vi "Viterbi.vi"(7 "Кадр с мягкими\nзначениями":dbl[](array[numeric])) -> (8 "Декодированный поток битов":bool[](array[boolean]))   [LabVIEW 2017]
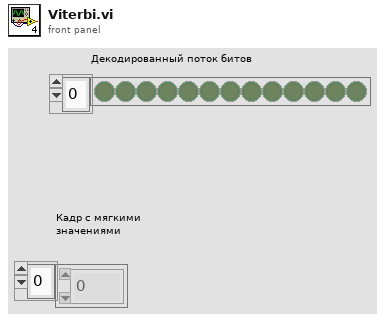
[diagram p1: front panel]
types:
  T1 = cluster{"Пр сост0":i32, "Ном зн\nреб0":i32, "Пр сост1":i32, "Ном зн\nреб1":i32, "Бит":bool}[]
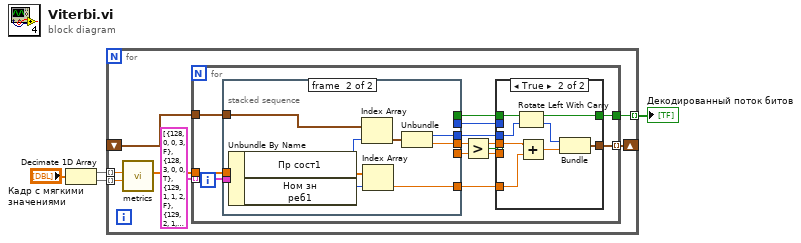
[diagram p0: block diagram]
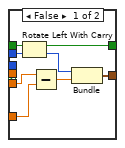
[diagram p2: hidden frame]
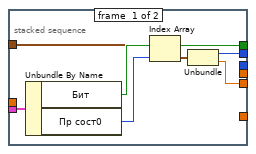
[diagram p3: hidden frame]
diagram:
  n1 = Decimate 1D Array("Кадр с мягкими\nзначениями") -> (w2:dbl[], w1:dbl[])
  n2 = for {
    tunnel: w2 -> [w10] mode=indexing
    tunnel: w1 -> [w9] mode=indexing
    tunnel: [w6] -> w3 mode=indexing
    shift-right: [w7] -> _
    shift-left: _ -> [w5]
    n3 = call "metrics.vi"("Бит неч"=w9, "Бит чет"=w10) -> ("Возможные\nметрики ребер"=w11:dbl[])  [unwired: 9 in]
    n4 = for {
      tunnel: T1 [{"Пр сост0"=128, "Ном зн\nреб0"=0, "Пр сост1"=0, "Ном зн\nреб1"=3, "Бит"=FALSE}, {"Пр сост0"=128, "Ном зн\nреб0"=3, "Пр сост1"=0, "Ном зн\nреб1"=0, "Бит"=TRUE}, {"Пр сост0"=129, "Ном зн\nреб0"=1, "Пр сост1"=1, "Ном зн\nреб1"=2, "Бит"=FALSE}, {"Пр сост0"=129, "Ном зн\nреб0"=2, "Пр сост1"=1, "Ном зн\nреб1"=1, "Бит"=TRUE}, {"Пр сост0"=130, "Ном зн\nреб0"=3, "Пр сост1"=2, "Ном зн\nреб1"=0, "Бит"=FALSE}, {"Пр сост0"=130, "Ном зн\nреб0"=0, "Пр сост1"=2, "Ном зн\nреб1"=3, "Бит"=TRUE}, {"Пр сост0"=131, "Ном зн\nреб0"=2, "Пр сост1"=3, "Ном зн\nреб1"=1, "Бит"=FALSE}, {"Пр сост0"=131, "Ном зн\nреб0"=1, "Пр сост1"=3, "Ном зн\nреб1"=2, "Бит"=TRUE}, {"Пр сост0"=132, "Ном зн\nреб0"=3, "Пр сост1"=4, "Ном зн\nреб1"=0, "Бит"=FALSE}, {"Пр сост0"=132, "Ном зн\nреб0"=0, "Пр сост1"=4, "Ном зн\nреб1"=3, "Бит"=TRUE}, {"Пр сост0"=133, "Ном зн\nреб0"=2, "Пр сост1"=5, "Ном зн\nреб1"=1, "Бит"=FALSE}, {"Пр сост0"=133, "Ном зн\nреб0"=1, "Пр сост1"=5, "Ном зн\nреб1"=2, "Бит"=TRUE}, {"Пр сост0"=134, "Ном зн\nреб0"=0, "Пр сост1"=6, "Ном зн\nреб1"=3, "Бит"=FALSE}, {"Пр сост0"=134, "Ном зн\nреб0"=3, "Пр сост1"=6, "Ном зн\nреб1"=0, "Бит"=TRUE}, {"Пр сост0"=135, "Ном зн\nреб0"=1, "Пр сост1"=7, "Ном зн\nреб1"=2, "Бит"=FALSE}, {"Пр сост0"=135, "Ном зн\nреб0"=2, "Пр сост1"=7, "Ном зн\nреб1"=1, "Бит"=TRUE}, {"Пр сост0"=136, "Ном зн\nреб0"=2, "Пр сост1"=8, "Ном зн\nреб1"=1, "Бит"=FALSE}, {"Пр сост0"=136, "Ном зн\nреб0"=1, "Пр сост1"=8, "Ном зн\nреб1"=2, "Бит"=TRUE}, {"Пр сост0"=137, "Ном зн\nреб0"=3, "Пр сост1"=9, "Ном зн\nреб1"=0, "Бит"=FALSE}, {"Пр сост0"=137, "Ном зн\nреб0"=0, "Пр сост1"=9, "Ном зн\nреб1"=3, "Бит"=TRUE}, {"Пр сост0"=138, "Ном зн\nреб0"=1, "Пр сост1"=10, "Ном зн\nреб1"=2, "Бит"=FALSE}, {"Пр сост0"=138, "Ном зн\nреб0"=2, "Пр сост1"=10, "Ном зн\nреб1"=1, "Бит"=TRUE}, {"Пр сост0"=139, "Ном зн\nреб0"=0, "Пр сост1"=11, "Ном зн\nреб1"=3, "Бит"=FALSE}, {"Пр сост0"=139, "Ном зн\nреб0"=3, "Пр сост1"=11, "Ном зн\nреб1"=0, "Бит"=TRUE}, {"Пр сост0"=140, "Ном зн\nреб0"=1, "Пр сост1"=12, "Ном зн\nреб1"=2, "Бит"=FALSE}, {"Пр сост0"=140, "Ном зн\nреб0"=2, "Пр сост1"=12, "Ном зн\nреб1"=1, "Бит"=TRUE}, {"Пр сост0"=141, "Ном зн\nреб0"=0, "Пр сост1"=13, "Ном зн\nреб1"=3, "Бит"=FALSE}, {"Пр сост0"=141, "Ном зн\nреб0"=3, "Пр сост1"=13, "Ном зн\nреб1"=0, "Бит"=TRUE}, {"Пр сост0"=142, "Ном зн\nреб0"=2, "Пр сост1"=14, "Ном зн\nреб1"=1, "Бит"=FALSE}, {"Пр сост0"=142, "Ном зн\nреб0"=1, "Пр сост1"=14, "Ном зн\nреб1"=2, "Бит"=TRUE}, {"Пр сост0"=143, "Ном зн\nреб0"=3, "Пр сост1"=15, "Ном зн\nреб1"=0, "Бит"=FALSE}, {"Пр сост0"=143, "Ном зн\nреб0"=0, "Пр сост1"=15, "Ном зн\nреб1"=3, "Бит"=TRUE}, {"Пр сост0"=144, "Ном зн\nреб0"=1, "Пр сост1"=16, "Ном зн\nреб1"=2, "Бит"=FALSE}, {"Пр сост0"=144, "Ном зн\nреб0"=2, "Пр сост1"=16, "Ном зн\nреб1"=1, "Бит"=TRUE}, {"Пр сост0"=145, "Ном зн\nреб0"=0, "Пр сост1"=17, "Ном зн\nреб1"=3, "Бит"=FALSE}, {"Пр сост0"=145, "Ном зн\nреб0"=3, "Пр сост1"=17, "Ном зн\nреб1"=0, "Бит"=TRUE}, {"Пр сост0"=146, "Ном зн\nреб0"=2, "Пр сост1"=18, "Ном зн\nреб1"=1, "Бит"=FALSE}, {"Пр сост0"=146, "Ном зн\nреб0"=1, "Пр сост1"=18, "Ном зн\nреб1"=2, "Бит"=TRUE}, {"Пр сост0"=147, "Ном зн\nреб0"=3, "Пр сост1"=19, "Ном зн\nреб1"=0, "Бит"=FALSE}, {"Пр сост0"=147, "Ном зн\nреб0"=0, "Пр сост1"=19, "Ном зн\nреб1"=3, "Бит"=TRUE}, {"Пр сост0"=148, "Ном зн\nреб0"=2, "Пр сост1"=20, "Ном зн\nреб1"=1, "Бит"=FALSE}, {"Пр сост0"=148, "Ном зн\nреб0"=1, "Пр сост1"=20, "Ном зн\nреб1"=2, "Бит"=TRUE}, {"Пр сост0"=149, "Ном зн\nреб0"=3, "Пр сост1"=21, "Ном зн\nреб1"=0, "Бит"=FALSE}, {"Пр сост0"=149, "Ном зн\nреб0"=0, "Пр сост1"=21, "Ном зн\nреб1"=3, "Бит"=TRUE}, {"Пр сост0"=150, "Ном зн\nреб0"=1, "Пр сост1"=22, "Ном зн\nреб1"=2, "Бит"=FALSE}, {"Пр сост0"=150, "Ном зн\nреб0"=2, "Пр сост1"=22, "Ном зн\nреб1"=1, "Бит"=TRUE}, {"Пр сост0"=151, "Ном зн\nреб0"=0, "Пр сост1"=23, "Ном зн\nреб1"=3, "Бит"=FALSE}, {"Пр сост0"=151, "Ном зн\nреб0"=3, "Пр сост1"=23, "Ном зн\nреб1"=0, "Бит"=TRUE}, {"Пр сост0"=152, "Ном зн\nреб0"=3, "Пр сост1"=24, "Ном зн\nреб1"=0, "Бит"=FALSE}, {"Пр сост0"=152, "Ном зн\nреб0"=0, "Пр сост1"=24, "Ном зн\nреб1"=3, "Бит"=TRUE}, {"Пр сост0"=153, "Ном зн\nреб0"=2, "Пр сост1"=25, "Ном зн\nреб1"=1, "Бит"=FALSE}, {"Пр сост0"=153, "Ном зн\nреб0"=1, "Пр сост1"=25, "Ном зн\nреб1"=2, "Бит"=TRUE}, {"Пр сост0"=154, "Ном зн\nреб0"=0, "Пр сост1"=26, "Ном зн\nреб1"=3, "Бит"=FALSE}, {"Пр сост0"=154, "Ном зн\nреб0"=3, "Пр сост1"=26, "Ном зн\nреб1"=0, "Бит"=TRUE}, {"Пр сост0"=155, "Ном зн\nреб0"=1, "Пр сост1"=27, "Ном зн\nреб1"=2, "Бит"=FALSE}, {"Пр сост0"=155, "Ном зн\nреб0"=2, "Пр сост1"=27, "Ном зн\nреб1"=1, "Бит"=TRUE}, {"Пр сост0"=156, "Ном зн\nреб0"=0, "Пр сост1"=28, "Ном зн\nреб1"=3, "Бит"=FALSE}, {"Пр сост0"=156, "Ном зн\nреб0"=3, "Пр сост1"=28, "Ном зн\nреб1"=0, "Бит"=TRUE}, {"Пр сост0"=157, "Ном зн\nреб0"=1, "Пр сост1"=29, "Ном зн\nреб1"=2, "Бит"=FALSE}, {"Пр сост0"=157, "Ном зн\nреб0"=2, "Пр сост1"=29, "Ном зн\nреб1"=1, "Бит"=TRUE}, {"Пр сост0"=158, "Ном зн\nреб0"=3, "Пр сост1"=30, "Ном зн\nреб1"=0, "Бит"=FALSE}, {"Пр сост0"=158, "Ном зн\nреб0"=0, "Пр сост1"=30, "Ном зн\nреб1"=3, "Бит"=TRUE}, {"Пр сост0"=159, "Ном зн\nреб0"=2, "Пр сост1"=31, "Ном зн\nреб1"=1, "Бит"=FALSE}, {"Пр сост0"=159, "Ном зн\nреб0"=1, "Пр сост1"=31, "Ном зн\nреб1"=2, "Бит"=TRUE}, {"Пр сост0"=160, "Ном зн\nреб0"=0, "Пр сост1"=32, "Ном зн\nреб1"=3, "Бит"=FALSE}, {"Пр сост0"=160, "Ном зн\nреб0"=3, "Пр сост1"=32, "Ном зн\nреб1"=0, "Бит"=TRUE}, {"Пр сост0"=161, "Ном зн\nреб0"=1, "Пр сост1"=33, "Ном зн\nреб1"=2, "Бит"=FALSE}, {"Пр сост0"=161, "Ном зн\nреб0"=2, "Пр сост1"=33, "Ном зн\nреб1"=1, "Бит"=TRUE}, {"Пр сост0"=162, "Ном зн\nреб0"=3, "Пр сост1"=34, "Ном зн\nреб1"=0, "Бит"=FALSE}, {"Пр сост0"=162, "Ном зн\nреб0"=0, "Пр сост1"=34, "Ном зн\nреб1"=3, "Бит"=TRUE}, {"Пр сост0"=163, "Ном зн\nреб0"=2, "Пр сост1"=35, "Ном зн\nреб1"=1, "Бит"=FALSE}, {"Пр сост0"=163, "Ном зн\nреб0"=1, "Пр сост1"=35, "Ном зн\nреб1"=2, "Бит"=TRUE}, {"Пр сост0"=164, "Ном зн\nреб0"=3, "Пр сост1"=36, "Ном зн\nреб1"=0, "Бит"=FALSE}, {"Пр сост0"=164, "Ном зн\nреб0"=0, "Пр сост1"=36, "Ном зн\nреб1"=3, "Бит"=TRUE}, {"Пр сост0"=165, "Ном зн\nреб0"=2, "Пр сост1"=37, "Ном зн\nреб1"=1, "Бит"=FALSE}, {"Пр сост0"=165, "Ном зн\nреб0"=1, "Пр сост1"=37, "Ном зн\nреб1"=2, "Бит"=TRUE}, {"Пр сост0"=166, "Ном зн\nреб0"=0, "Пр сост1"=38, "Ном зн\nреб1"=3, "Бит"=FALSE}, {"Пр сост0"=166, "Ном зн\nреб0"=3, "Пр сост1"=38, "Ном зн\nреб1"=0, "Бит"=TRUE}, {"Пр сост0"=167, "Ном зн\nреб0"=1, "Пр сост1"=39, "Ном зн\nреб1"=2, "Бит"=FALSE}, {"Пр сост0"=167, "Ном зн\nреб0"=2, "Пр сост1"=39, "Ном зн\nреб1"=1, "Бит"=TRUE}, {"Пр сост0"=168, "Ном зн\nреб0"=2, "Пр сост1"=40, "Ном зн\nреб1"=1, "Бит"=FALSE}, {"Пр сост0"=168, "Ном зн\nреб0"=1, "Пр сост1"=40, "Ном зн\nреб1"=2, "Бит"=TRUE}, {"Пр сост0"=169, "Ном зн\nреб0"=3, "Пр сост1"=41, "Ном зн\nреб1"=0, "Бит"=FALSE}, {"Пр сост0"=169, "Ном зн\nреб0"=0, "Пр сост1"=41, "Ном зн\nреб1"=3, "Бит"=TRUE}, {"Пр сост0"=170, "Ном зн\nреб0"=1, "Пр сост1"=42, "Ном зн\nреб1"=2, "Бит"=FALSE}, {"Пр сост0"=170, "Ном зн\nреб0"=2, "Пр сост1"=42, "Ном зн\nреб1"=1, "Бит"=TRUE}, {"Пр сост0"=171, "Ном зн\nреб0"=0, "Пр сост1"=43, "Ном зн\nреб1"=3, "Бит"=FALSE}, {"Пр сост0"=171, "Ном зн\nреб0"=3, "Пр сост1"=43, "Ном зн\nреб1"=0, "Бит"=TRUE}, {"Пр сост0"=172, "Ном зн\nреб0"=1, "Пр сост1"=44, "Ном зн\nреб1"=2, "Бит"=FALSE}, {"Пр сост0"=172, "Ном зн\nреб0"=2, "Пр сост1"=44, "Ном зн\nреб1"=1, "Бит"=TRUE}, {"Пр сост0"=173, "Ном зн\nреб0"=0, "Пр сост1"=45, "Ном зн\nреб1"=3, "Бит"=FALSE}, {"Пр сост0"=173, "Ном зн\nреб0"=3, "Пр сост1"=45, "Ном зн\nреб1"=0, "Бит"=TRUE}, {"Пр сост0"=174, "Ном зн\nреб0"=2, "Пр сост1"=46, "Ном зн\nреб1"=1, "Бит"=FALSE}, {"Пр сост0"=174, "Ном зн\nреб0"=1, "Пр сост1"=46, "Ном зн\nреб1"=2, "Бит"=TRUE}, {"Пр сост0"=175, "Ном зн\nреб0"=3, "Пр сост1"=47, "Ном зн\nреб1"=0, "Бит"=FALSE}, {"Пр сост0"=175, "Ном зн\nреб0"=0, "Пр сост1"=47, "Ном зн\nреб1"=3, "Бит"=TRUE}, {"Пр сост0"=176, "Ном зн\nреб0"=1, "Пр сост1"=48, "Ном зн\nреб1"=2, "Бит"=FALSE}, {"Пр сост0"=176, "Ном зн\nреб0"=2, "Пр сост1"=48, "Ном зн\nреб1"=1, "Бит"=TRUE}, {"Пр сост0"=177, "Ном зн\nреб0"=0, "Пр сост1"=49, "Ном зн\nреб1"=3, "Бит"=FALSE}, {"Пр сост0"=177, "Ном зн\nреб0"=3, "Пр сост1"=49, "Ном зн\nреб1"=0, "Бит"=TRUE}, {"Пр сост0"=178, "Ном зн\nреб0"=2, "Пр сост1"=50, "Ном зн\nреб1"=1, "Бит"=FALSE}, {"Пр сост0"=178, "Ном зн\nреб0"=1, "Пр сост1"=50, "Ном зн\nреб1"=2, "Бит"=TRUE}, {"Пр сост0"=179, "Ном зн\nреб0"=3, "Пр сост1"=51, "Ном зн\nреб1"=0, "Бит"=FALSE}, {"Пр сост0"=179, "Ном зн\nреб0"=0, "Пр сост1"=51, "Ном зн\nреб1"=3, "Бит"=TRUE}, {"Пр сост0"=180, "Ном зн\nреб0"=2, "Пр сост1"=52, "Ном зн\nреб1"=1, "Бит"=FALSE}, {"Пр сост0"=180, "Ном зн\nреб0"=1, "Пр сост1"=52, "Ном зн\nреб1"=2, "Бит"=TRUE}, {"Пр сост0"=181, "Ном зн\nреб0"=3, "Пр сост1"=53, "Ном зн\nреб1"=0, "Бит"=FALSE}, {"Пр сост0"=181, "Ном зн\nреб0"=0, "Пр сост1"=53, "Ном зн\nреб1"=3, "Бит"=TRUE}, {"Пр сост0"=182, "Ном зн\nреб0"=1, "Пр сост1"=54, "Ном зн\nреб1"=2, "Бит"=FALSE}, {"Пр сост0"=182, "Ном зн\nреб0"=2, "Пр сост1"=54, "Ном зн\nреб1"=1, "Бит"=TRUE}, {"Пр сост0"=183, "Ном зн\nреб0"=0, "Пр сост1"=55, "Ном зн\nреб1"=3, "Бит"=FALSE}, {"Пр сост0"=183, "Ном зн\nреб0"=3, "Пр сост1"=55, "Ном зн\nреб1"=0, "Бит"=TRUE}, {"Пр сост0"=184, "Ном зн\nреб0"=3, "Пр сост1"=56, "Ном зн\nреб1"=0, "Бит"=FALSE}, {"Пр сост0"=184, "Ном зн\nреб0"=0, "Пр сост1"=56, "Ном зн\nреб1"=3, "Бит"=TRUE}, {"Пр сост0"=185, "Ном зн\nреб0"=2, "Пр сост1"=57, "Ном зн\nреб1"=1, "Бит"=FALSE}, {"Пр сост0"=185, "Ном зн\nреб0"=1, "Пр сост1"=57, "Ном зн\nреб1"=2, "Бит"=TRUE}, {"Пр сост0"=186, "Ном зн\nреб0"=0, "Пр сост1"=58, "Ном зн\nреб1"=3, "Бит"=FALSE}, {"Пр сост0"=186, "Ном зн\nреб0"=3, "Пр сост1"=58, "Ном зн\nреб1"=0, "Бит"=TRUE}, {"Пр сост0"=187, "Ном зн\nреб0"=1, "Пр сост1"=59, "Ном зн\nреб1"=2, "Бит"=FALSE}, {"Пр сост0"=187, "Ном зн\nреб0"=2, "Пр сост1"=59, "Ном зн\nреб1"=1, "Бит"=TRUE}, {"Пр сост0"=188, "Ном зн\nреб0"=0, "Пр сост1"=60, "Ном зн\nреб1"=3, "Бит"=FALSE}, {"Пр сост0"=188, "Ном зн\nреб0"=3, "Пр сост1"=60, "Ном зн\nреб1"=0, "Бит"=TRUE}, {"Пр сост0"=189, "Ном зн\nреб0"=1, "Пр сост1"=61, "Ном зн\nреб1"=2, "Бит"=FALSE}, {"Пр сост0"=189, "Ном зн\nреб0"=2, "Пр сост1"=61, "Ном зн\nреб1"=1, "Бит"=TRUE}, {"Пр сост0"=190, "Ном зн\nреб0"=3, "Пр сост1"=62, "Ном зн\nреб1"=0, "Бит"=FALSE}, {"Пр сост0"=190, "Ном зн\nреб0"=0, "Пр сост1"=62, "Ном зн\nреб1"=3, "Бит"=TRUE}, {"Пр сост0"=191, "Ном зн\nреб0"=2, "Пр сост1"=63, "Ном зн\nреб1"=1, "Бит"=FALSE}, {"Пр сост0"=191, "Ном зн\nреб0"=1, "Пр сост1"=63, "Ном зн\nреб1"=2, "Бит"=TRUE}, {"Пр сост0"=192, "Ном зн\nреб0"=1, "Пр сост1"=64, "Ном зн\nреб1"=2, "Бит"=FALSE}, {"Пр сост0"=192, "Ном зн\nреб0"=2, "Пр сост1"=64, "Ном зн\nреб1"=1, "Бит"=TRUE}, {"Пр сост0"=193, "Ном зн\nреб0"=0, "Пр сост1"=65, "Ном зн\nреб1"=3, "Бит"=FALSE}, {"Пр сост0"=193, "Ном зн\nреб0"=3, "Пр сост1"=65, "Ном зн\nреб1"=0, "Бит"=TRUE}, {"Пр сост0"=194, "Ном зн\nреб0"=2, "Пр сост1"=66, "Ном зн\nреб1"=1, "Бит"=FALSE}, {"Пр сост0"=194, "Ном зн\nреб0"=1, "Пр сост1"=66, "Ном зн\nреб1"=2, "Бит"=TRUE}, {"Пр сост0"=195, "Ном зн\nреб0"=3, "Пр сост1"=67, "Ном зн\nреб1"=0, "Бит"=FALSE}, {"Пр сост0"=195, "Ном зн\nреб0"=0, "Пр сост1"=67, "Ном зн\nреб1"=3, "Бит"=TRUE}, {"Пр сост0"=196, "Ном зн\nреб0"=2, "Пр сост1"=68, "Ном зн\nреб1"=1, "Бит"=FALSE}, {"Пр сост0"=196, "Ном зн\nреб0"=1, "Пр сост1"=68, "Ном зн\nреб1"=2, "Бит"=TRUE}, {"Пр сост0"=197, "Ном зн\nреб0"=3, "Пр сост1"=69, "Ном зн\nреб1"=0, "Бит"=FALSE}, {"Пр сост0"=197, "Ном зн\nреб0"=0, "Пр сост1"=69, "Ном зн\nреб1"=3, "Бит"=TRUE}, {"Пр сост0"=198, "Ном зн\nреб0"=1, "Пр сост1"=70, "Ном зн\nреб1"=2, "Бит"=FALSE}, {"Пр сост0"=198, "Ном зн\nреб0"=2, "Пр сост1"=70, "Ном зн\nреб1"=1, "Бит"=TRUE}, {"Пр сост0"=199, "Ном зн\nреб0"=0, "Пр сост1"=71, "Ном зн\nреб1"=3, "Бит"=FALSE}, {"Пр сост0"=199, "Ном зн\nреб0"=3, "Пр сост1"=71, "Ном зн\nреб1"=0, "Бит"=TRUE}, {"Пр сост0"=200, "Ном зн\nреб0"=3, "Пр сост1"=72, "Ном зн\nреб1"=0, "Бит"=FALSE}, {"Пр сост0"=200, "Ном зн\nреб0"=0, "Пр сост1"=72, "Ном зн\nреб1"=3, "Бит"=TRUE}, {"Пр сост0"=201, "Ном зн\nреб0"=2, "Пр сост1"=73, "Ном зн\nреб1"=1, "Бит"=FALSE}, {"Пр сост0"=201, "Ном зн\nреб0"=1, "Пр сост1"=73, "Ном зн\nреб1"=2, "Бит"=TRUE}, {"Пр сост0"=202, "Ном зн\nреб0"=0, "Пр сост1"=74, "Ном зн\nреб1"=3, "Бит"=FALSE}, {"Пр сост0"=202, "Ном зн\nреб0"=3, "Пр сост1"=74, "Ном зн\nреб1"=0, "Бит"=TRUE}, {"Пр сост0"=203, "Ном зн\nреб0"=1, "Пр сост1"=75, "Ном зн\nреб1"=2, "Бит"=FALSE}, {"Пр сост0"=203, "Ном зн\nреб0"=2, "Пр сост1"=75, "Ном зн\nреб1"=1, "Бит"=TRUE}, {"Пр сост0"=204, "Ном зн\nреб0"=0, "Пр сост1"=76, "Ном зн\nреб1"=3, "Бит"=FALSE}, {"Пр сост0"=204, "Ном зн\nреб0"=3, "Пр сост1"=76, "Ном зн\nреб1"=0, "Бит"=TRUE}, {"Пр сост0"=205, "Ном зн\nреб0"=1, "Пр сост1"=77, "Ном зн\nреб1"=2, "Бит"=FALSE}, {"Пр сост0"=205, "Ном зн\nреб0"=2, "Пр сост1"=77, "Ном зн\nреб1"=1, "Бит"=TRUE}, {"Пр сост0"=206, "Ном зн\nреб0"=3, "Пр сост1"=78, "Ном зн\nреб1"=0, "Бит"=FALSE}, {"Пр сост0"=206, "Ном зн\nреб0"=0, "Пр сост1"=78, "Ном зн\nреб1"=3, "Бит"=TRUE}, {"Пр сост0"=207, "Ном зн\nреб0"=2, "Пр сост1"=79, "Ном зн\nреб1"=1, "Бит"=FALSE}, {"Пр сост0"=207, "Ном зн\nреб0"=1, "Пр сост1"=79, "Ном зн\nреб1"=2, "Бит"=TRUE}, {"Пр сост0"=208, "Ном зн\nреб0"=0, "Пр сост1"=80, "Ном зн\nреб1"=3, "Бит"=FALSE}, {"Пр сост0"=208, "Ном зн\nреб0"=3, "Пр сост1"=80, "Ном зн\nреб1"=0, "Бит"=TRUE}, {"Пр сост0"=209, "Ном зн\nреб0"=1, "Пр сост1"=81, "Ном зн\nреб1"=2, "Бит"=FALSE}, {"Пр сост0"=209, "Ном зн\nреб0"=2, "Пр сост1"=81, "Ном зн\nреб1"=1, "Бит"=TRUE}, {"Пр сост0"=210, "Ном зн\nреб0"=3, "Пр сост1"=82, "Ном зн\nреб1"=0, "Бит"=FALSE}, {"Пр сост0"=210, "Ном зн\nреб0"=0, "Пр сост1"=82, "Ном зн\nреб1"=3, "Бит"=TRUE}, {"Пр сост0"=211, "Ном зн\nреб0"=2, "Пр сост1"=83, "Ном зн\nреб1"=1, "Бит"=FALSE}, {"Пр сост0"=211, "Ном зн\nреб0"=1, "Пр сост1"=83, "Ном зн\nреб1"=2, "Бит"=TRUE}, {"Пр сост0"=212, "Ном зн\nреб0"=3, "Пр сост1"=84, "Ном зн\nреб1"=0, "Бит"=FALSE}, {"Пр сост0"=212, "Ном зн\nреб0"=0, "Пр сост1"=84, "Ном зн\nреб1"=3, "Бит"=TRUE}, {"Пр сост0"=213, "Ном зн\nреб0"=2, "Пр сост1"=85, "Ном зн\nреб1"=1, "Бит"=FALSE}, {"Пр сост0"=213, "Ном зн\nреб0"=1, "Пр сост1"=85, "Ном зн\nреб1"=2, "Бит"=TRUE}, {"Пр сост0"=214, "Ном зн\nреб0"=0, "Пр сост1"=86, "Ном зн\nреб1"=3, "Бит"=FALSE}, {"Пр сост0"=214, "Ном зн\nреб0"=3, "Пр сост1"=86, "Ном зн\nреб1"=0, "Бит"=TRUE}, {"Пр сост0"=215, "Ном зн\nреб0"=1, "Пр сост1"=87, "Ном зн\nреб1"=2, "Бит"=FALSE}, {"Пр сост0"=215, "Ном зн\nреб0"=2, "Пр сост1"=87, "Ном зн\nреб1"=1, "Бит"=TRUE}, {"Пр сост0"=216, "Ном зн\nреб0"=2, "Пр сост1"=88, "Ном зн\nреб1"=1, "Бит"=FALSE}, {"Пр сост0"=216, "Ном зн\nреб0"=1, "Пр сост1"=88, "Ном зн\nреб1"=2, "Бит"=TRUE}, {"Пр сост0"=217, "Ном зн\nреб0"=3, "Пр сост1"=89, "Ном зн\nреб1"=0, "Бит"=FALSE}, {"Пр сост0"=217, "Ном зн\nреб0"=0, "Пр сост1"=89, "Ном зн\nреб1"=3, "Бит"=TRUE}, {"Пр сост0"=218, "Ном зн\nреб0"=1, "Пр сост1"=90, "Ном зн\nреб1"=2, "Бит"=FALSE}, {"Пр сост0"=218, "Ном зн\nреб0"=2, "Пр сост1"=90, "Ном зн\nреб1"=1, "Бит"=TRUE}, {"Пр сост0"=219, "Ном зн\nреб0"=0, "Пр сост1"=91, "Ном зн\nреб1"=3, "Бит"=FALSE}, {"Пр сост0"=219, "Ном зн\nреб0"=3, "Пр сост1"=91, "Ном зн\nреб1"=0, "Бит"=TRUE}, {"Пр сост0"=220, "Ном зн\nреб0"=1, "Пр сост1"=92, "Ном зн\nреб1"=2, "Бит"=FALSE}, {"Пр сост0"=220, "Ном зн\nреб0"=2, "Пр сост1"=92, "Ном зн\nреб1"=1, "Бит"=TRUE}, {"Пр сост0"=221, "Ном зн\nреб0"=0, "Пр сост1"=93, "Ном зн\nреб1"=3, "Бит"=FALSE}, {"Пр сост0"=221, "Ном зн\nреб0"=3, "Пр сост1"=93, "Ном зн\nреб1"=0, "Бит"=TRUE}, {"Пр сост0"=222, "Ном зн\nреб0"=2, "Пр сост1"=94, "Ном зн\nреб1"=1, "Бит"=FALSE}, {"Пр сост0"=222, "Ном зн\nреб0"=1, "Пр сост1"=94, "Ном зн\nреб1"=2, "Бит"=TRUE}, {"Пр сост0"=223, "Ном зн\nреб0"=3, "Пр сост1"=95, "Ном зн\nреб1"=0, "Бит"=FALSE}, {"Пр сост0"=223, "Ном зн\nреб0"=0, "Пр сост1"=95, "Ном зн\nреб1"=3, "Бит"=TRUE}, {"Пр сост0"=224, "Ном зн\nреб0"=1, "Пр сост1"=96, "Ном зн\nреб1"=2, "Бит"=FALSE}, {"Пр сост0"=224, "Ном зн\nреб0"=2, "Пр сост1"=96, "Ном зн\nреб1"=1, "Бит"=TRUE}, {"Пр сост0"=225, "Ном зн\nреб0"=0, "Пр сост1"=97, "Ном зн\nреб1"=3, "Бит"=FALSE}, {"Пр сост0"=225, "Ном зн\nреб0"=3, "Пр сост1"=97, "Ном зн\nреб1"=0, "Бит"=TRUE}, {"Пр сост0"=226, "Ном зн\nреб0"=2, "Пр сост1"=98, "Ном зн\nреб1"=1, "Бит"=FALSE}, {"Пр сост0"=226, "Ном зн\nреб0"=1, "Пр сост1"=98, "Ном зн\nреб1"=2, "Бит"=TRUE}, {"Пр сост0"=227, "Ном зн\nреб0"=3, "Пр сост1"=99, "Ном зн\nреб1"=0, "Бит"=FALSE}, {"Пр сост0"=227, "Ном зн\nреб0"=0, "Пр сост1"=99, "Ном зн\nреб1"=3, "Бит"=TRUE}, {"Пр сост0"=228, "Ном зн\nреб0"=2, "Пр сост1"=100, "Ном зн\nреб1"=1, "Бит"=FALSE}, {"Пр сост0"=228, "Ном зн\nреб0"=1, "Пр сост1"=100, "Ном зн\nреб1"=2, "Бит"=TRUE}, {"Пр сост0"=229, "Ном зн\nреб0"=3, "Пр сост1"=101, "Ном зн\nреб1"=0, "Бит"=FALSE}, {"Пр сост0"=229, "Ном зн\nреб0"=0, "Пр сост1"=101, "Ном зн\nреб1"=3, "Бит"=TRUE}, {"Пр сост0"=230, "Ном зн\nреб0"=1, "Пр сост1"=102, "Ном зн\nреб1"=2, "Бит"=FALSE}, {"Пр сост0"=230, "Ном зн\nреб0"=2, "Пр сост1"=102, "Ном зн\nреб1"=1, "Бит"=TRUE}, {"Пр сост0"=231, "Ном зн\nреб0"=0, "Пр сост1"=103, "Ном зн\nреб1"=3, "Бит"=FALSE}, {"Пр сост0"=231, "Ном зн\nреб0"=3, "Пр сост1"=103, "Ном зн\nреб1"=0, "Бит"=TRUE}, {"Пр сост0"=232, "Ном зн\nреб0"=3, "Пр сост1"=104, "Ном зн\nреб1"=0, "Бит"=FALSE}, {"Пр сост0"=232, "Ном зн\nреб0"=0, "Пр сост1"=104, "Ном зн\nреб1"=3, "Бит"=TRUE}, {"Пр сост0"=233, "Ном зн\nреб0"=2, "Пр сост1"=105, "Ном зн\nреб1"=1, "Бит"=FALSE}, {"Пр сост0"=233, "Ном зн\nреб0"=1, "Пр сост1"=105, "Ном зн\nреб1"=2, "Бит"=TRUE}, {"Пр сост0"=234, "Ном зн\nреб0"=0, "Пр сост1"=106, "Ном зн\nреб1"=3, "Бит"=FALSE}, {"Пр сост0"=234, "Ном зн\nреб0"=3, "Пр сост1"=106, "Ном зн\nреб1"=0, "Бит"=TRUE}, {"Пр сост0"=235, "Ном зн\nреб0"=1, "Пр сост1"=107, "Ном зн\nреб1"=2, "Бит"=FALSE}, {"Пр сост0"=235, "Ном зн\nреб0"=2, "Пр сост1"=107, "Ном зн\nреб1"=1, "Бит"=TRUE}, {"Пр сост0"=236, "Ном зн\nреб0"=0, "Пр сост1"=108, "Ном зн\nреб1"=3, "Бит"=FALSE}, {"Пр сост0"=236, "Ном зн\nреб0"=3, "Пр сост1"=108, "Ном зн\nреб1"=0, "Бит"=TRUE}, {"Пр сост0"=237, "Ном зн\nреб0"=1, "Пр сост1"=109, "Ном зн\nреб1"=2, "Бит"=FALSE}, {"Пр сост0"=237, "Ном зн\nреб0"=2, "Пр сост1"=109, "Ном зн\nреб1"=1, "Бит"=TRUE}, {"Пр сост0"=238, "Ном зн\nреб0"=3, "Пр сост1"=110, "Ном зн\nреб1"=0, "Бит"=FALSE}, {"Пр сост0"=238, "Ном зн\nреб0"=0, "Пр сост1"=110, "Ном зн\nреб1"=3, "Бит"=TRUE}, {"Пр сост0"=239, "Ном зн\nреб0"=2, "Пр сост1"=111, "Ном зн\nреб1"=1, "Бит"=FALSE}, {"Пр сост0"=239, "Ном зн\nреб0"=1, "Пр сост1"=111, "Ном зн\nреб1"=2, "Бит"=TRUE}, {"Пр сост0"=240, "Ном зн\nреб0"=0, "Пр сост1"=112, "Ном зн\nреб1"=3, "Бит"=FALSE}, {"Пр сост0"=240, "Ном зн\nреб0"=3, "Пр сост1"=112, "Ном зн\nреб1"=0, "Бит"=TRUE}, {"Пр сост0"=241, "Ном зн\nреб0"=1, "Пр сост1"=113, "Ном зн\nреб1"=2, "Бит"=FALSE}, {"Пр сост0"=241, "Ном зн\nреб0"=2, "Пр сост1"=113, "Ном зн\nреб1"=1, "Бит"=TRUE}, {"Пр сост0"=242, "Ном зн\nреб0"=3, "Пр сост1"=114, "Ном зн\nреб1"=0, "Бит"=FALSE}, {"Пр сост0"=242, "Ном зн\nреб0"=0, "Пр сост1"=114, "Ном зн\nреб1"=3, "Бит"=TRUE}, {"Пр сост0"=243, "Ном зн\nреб0"=2, "Пр сост1"=115, "Ном зн\nреб1"=1, "Бит"=FALSE}, {"Пр сост0"=243, "Ном зн\nреб0"=1, "Пр сост1"=115, "Ном зн\nреб1"=2, "Бит"=TRUE}, {"Пр сост0"=244, "Ном зн\nреб0"=3, "Пр сост1"=116, "Ном зн\nреб1"=0, "Бит"=FALSE}, {"Пр сост0"=244, "Ном зн\nреб0"=0, "Пр сост1"=116, "Ном зн\nреб1"=3, "Бит"=TRUE}, {"Пр сост0"=245, "Ном зн\nреб0"=2, "Пр сост1"=117, "Ном зн\nреб1"=1, "Бит"=FALSE}, {"Пр сост0"=245, "Ном зн\nреб0"=1, "Пр сост1"=117, "Ном зн\nреб1"=2, "Бит"=TRUE}, {"Пр сост0"=246, "Ном зн\nреб0"=0, "Пр сост1"=118, "Ном зн\nреб1"=3, "Бит"=FALSE}, {"Пр сост0"=246, "Ном зн\nреб0"=3, "Пр сост1"=118, "Ном зн\nреб1"=0, "Бит"=TRUE}, {"Пр сост0"=247, "Ном зн\nреб0"=1, "Пр сост1"=119, "Ном зн\nреб1"=2, "Бит"=FALSE}, {"Пр сост0"=247, "Ном зн\nреб0"=2, "Пр сост1"=119, "Ном зн\nреб1"=1, "Бит"=TRUE}, {"Пр сост0"=248, "Ном зн\nреб0"=2, "Пр сост1"=120, "Ном зн\nреб1"=1, "Бит"=FALSE}, {"Пр сост0"=248, "Ном зн\nреб0"=1, "Пр сост1"=120, "Ном зн\nреб1"=2, "Бит"=TRUE}, {"Пр сост0"=249, "Ном зн\nреб0"=3, "Пр сост1"=121, "Ном зн\nреб1"=0, "Бит"=FALSE}, {"Пр сост0"=249, "Ном зн\nреб0"=0, "Пр сост1"=121, "Ном зн\nреб1"=3, "Бит"=TRUE}, {"Пр сост0"=250, "Ном зн\nреб0"=1, "Пр сост1"=122, "Ном зн\nреб1"=2, "Бит"=FALSE}, {"Пр сост0"=250, "Ном зн\nреб0"=2, "Пр сост1"=122, "Ном зн\nреб1"=1, "Бит"=TRUE}, {"Пр сост0"=251, "Ном зн\nреб0"=0, "Пр сост1"=123, "Ном зн\nреб1"=3, "Бит"=FALSE}, {"Пр сост0"=251, "Ном зн\nреб0"=3, "Пр сост1"=123, "Ном зн\nреб1"=0, "Бит"=TRUE}, {"Пр сост0"=252, "Ном зн\nреб0"=1, "Пр сост1"=124, "Ном зн\nреб1"=2, "Бит"=FALSE}, {"Пр сост0"=252, "Ном зн\nреб0"=2, "Пр сост1"=124, "Ном зн\nреб1"=1, "Бит"=TRUE}, {"Пр сост0"=253, "Ном зн\nреб0"=0, "Пр сост1"=125, "Ном зн\nреб1"=3, "Бит"=FALSE}, {"Пр сост0"=253, "Ном зн\nреб0"=3, "Пр сост1"=125, "Ном зн\nреб1"=0, "Бит"=TRUE}, {"Пр сост0"=254, "Ном зн\nреб0"=2, "Пр сост1"=126, "Ном зн\nреб1"=1, "Бит"=FALSE}, {"Пр сост0"=254, "Ном зн\nреб0"=1, "Пр сост1"=126, "Ном зн\nреб1"=2, "Бит"=TRUE}, {"Пр сост0"=255, "Ном зн\nреб0"=3, "Пр сост1"=127, "Ном зн\nреб1"=0, "Бит"=FALSE}, {"Пр сост0"=255, "Ном зн\nреб0"=0, "Пр сост1"=127, "Ном зн\nреб1"=3, "Бит"=TRUE}] ("Параметры метрики 2") -> [w23] mode=indexing
      tunnel: w11 -> [w22]
      tunnel: [w19] -> w6
      tunnel: [w17] -> w7 mode=indexing
      tunnel: w5 -> [w16]
      n5 = stacked-sequence {
        tunnel: w23 -> [w46 w53]
        tunnel: w22 -> [_ w54]
        tunnel: [w40 _] -> w13
        tunnel: [_ w48] -> w18
        tunnel: [w45 _] -> w20
        tunnel: w16 -> [w44 w51]
        tunnel: [w41 _] -> w15
        tunnel: [_ w49] -> w14
        tunnel: [_ w47] -> w12
        frame #0 {
          n6 = Unbundle By Name(w46) -> ("Бит"=w45:bool, "Пр сост0"=w43:i32)
          n7 = Index Array(array=w44, index=w43) -> (element=w42:cluster{u64, dbl})
          n8 = Unbundle(w42) -> (w41:u64, w40:dbl)
        }
        frame #1 {
          n9 = Unbundle By Name(w53) -> ("Пр сост1"=w50:i32, "Ном зн\nреб1"=w55:i32)
          n10 = Index Array(array=w51, index=w50) -> (element=w52:cluster{u64, dbl})
          n11 = Index Array(array=w54, index=w55) -> (element=w47:dbl)
          n12 = Unbundle(w52) -> (w49:u64, w48:dbl)
        }
      }
      n13 = Greater?(x=w18, y=w13) -> (0:w21:bool)
      n14 = case shown="True" w21 {
        tunnel: w20 -> [w30 w39]
        tunnel: [w29 w38] -> w19
        tunnel: w18 -> [_ w34]
        tunnel: [w28 w36] -> w17
        tunnel: w13 -> [w26 _]
        tunnel: w15 -> [w27 _]
        tunnel: w14 -> [_ w35]
        tunnel: w12 -> [w24 w33]
        frame False {
          n15 = Rotate Left With Carry(2:w27, 3:w30) -> (0:w31:u64, 1:w29:bool)
          n16 = Subtract(x=w26, y=w24) -> (x-y=w25:dbl)
          n17 = Bundle(w31, w25) -> (w28:cluster{u64, dbl})  [unwired: 1 in]
        }
        frame True {
          n18 = Rotate Left With Carry(2:w35, 3:w39) -> (0:w37:u64, 1:w38:bool)
          n19 = Add(x=w34, y=w33) -> (x+y=w32:dbl)
          n20 = Bundle(w37, w32) -> (w36:cluster{u64, dbl})  [unwired: 1 in]
        }
      }
    }
  }
  "Декодированный поток битов" <- w3
